vi "Get Elements.vi"(8 "error in (no error)":errorcluster, 10 "Keys (empty: All)":string[](array[string]), 11 "SMO.Dictionary.Variant in":refnum<class "SMO.Dictionary.Variant.lvclass">) -> (0 "error out":errorcluster, 1 "Values":variant[](array[variant]), 2 "Keys out":string[](array[string]), 3 "SMO.Dictionary.Variant out":refnum<class "SMO.Dictionary.Variant.lvclass">)   [LabVIEW 2013, in "SMO.Dictionary.lvlib" / "SMO.Dictionary.Variant.lvclass"]
uses:
  SMO.Dictionary.Variant.lvclass
  SMO.Dictionary.Variant.lvclass/SMO.Dictionary.Variant.ctl
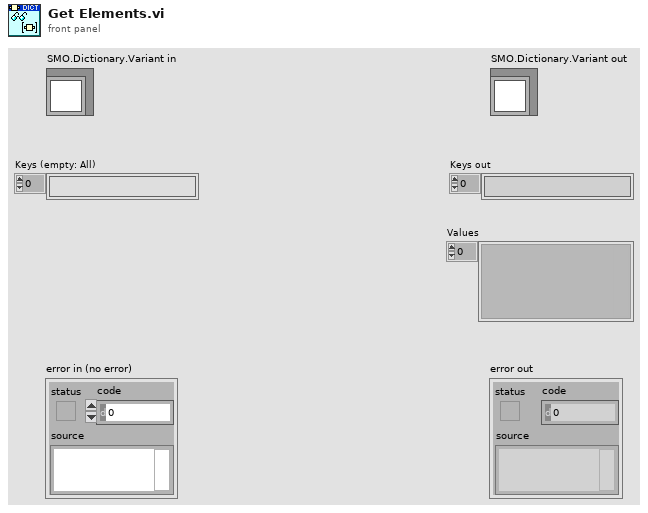
[diagram p1: front panel]
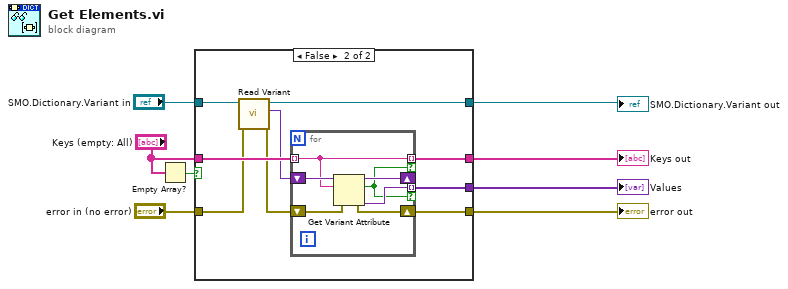
[diagram p0: block diagram]
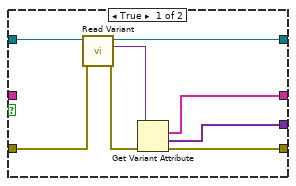
[diagram p2: hidden frame]
diagram:
  n1 = Empty Array?(array="Keys (empty: All)") -> (empty?=w4:bool)
  n2 = case shown="False" w4 {
    tunnel: "SMO.Dictionary.Variant in" -> [w13 w21]
    tunnel: [w14 w22] -> w7
    tunnel: [w9 w19] -> w6
    tunnel: "error in (no error)" -> [w11 w18]
    tunnel: [w16 w23] -> w3
    tunnel: [w15 w25] -> w2
    tunnel: "Keys (empty: All)" -> [_ w24]
    frame True {
      n3 = call "Read Variant.vi"("error in (no error)"=w11, "SMO.Dictionary.Variant in"=w13) -> ("error out"=w10:errorcluster, "Variant"=w12:variant, "SMO.Dictionary.Variant out"=w14:refnum<class "SMO.Dictionary.Variant.lvclass">)  [unwired: 7 in]
      n4 = Get Variant Attribute(Variant=w12, error in=w10) -> (names=w16:string[], values=w15:variant[], error out=w9:errorcluster)  [unwired: 2 in, 1 out]
    }
    frame False {
      n5 = call "Read Variant.vi"("error in (no error)"=w18, "SMO.Dictionary.Variant in"=w21) -> ("error out"=w17:errorcluster, "Variant"=w20:variant, "SMO.Dictionary.Variant out"=w22:refnum<class "SMO.Dictionary.Variant.lvclass">)  [unwired: 7 in]
      n6 = for {
        tunnel: [w28] -> w25 mode=indexing if=w27
        tunnel: w24 -> [w26] mode=indexing
        tunnel: [w26] -> w23 mode=indexing if=w27
        shift-right: [w30] -> w19
        shift-left: w17 -> [w29]
        shift-right: [w31] -> _
        shift-left: w20 -> [w32]
        n7 = Get Variant Attribute(Variant=w32, name=w26, error in=w29) -> (duplicate Variant=w31:variant, found=w27:bool, value=w28:variant, error out=w30:errorcluster)  [unwired: 1 in]
      }
    }
  }
  "error out" <- w6
  "SMO.Dictionary.Variant out" <- w7
  "Values" <- w2
  "Keys out" <- w3
